vi "add datafile(SubVI).vi"(10 "字符串":string) -> (1 "ok or cancel":bool=TRUE, 2 "连接的字符串":string)   [LabVIEW 2019, in "Add Seq.lvlib"]
uses:
  Add Seq.lvlib
panel:
  in  "cancel":bool
  in  "ok":bool
  in  "operation(0:open)":T1(ring)=enum."create"
  in  "path":path
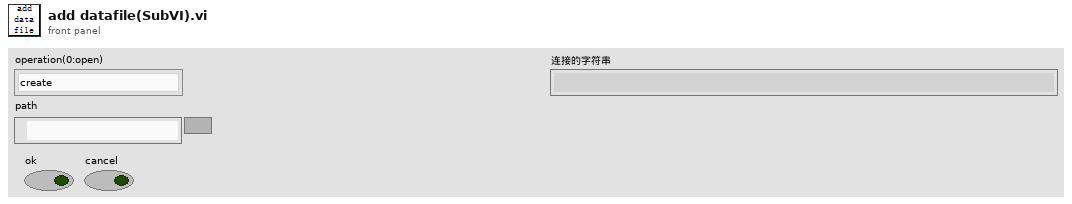
[diagram p1: front panel]
types:
  T1 = enum16{"open", "replace", "create", "open or create", "replace or create"}
  T2 = enum16{"open", "replace", "create", "open or create", "replace or create", "replace or create with confirmation"}
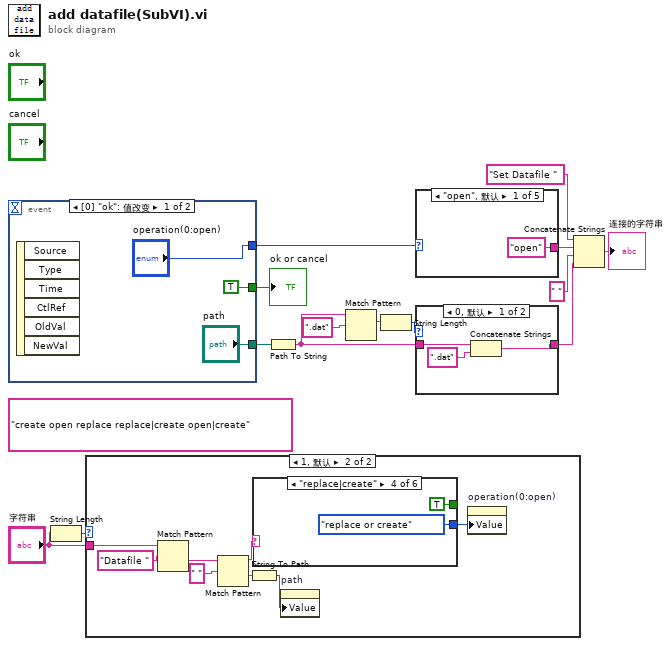
[diagram p0: block diagram]
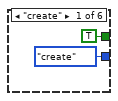
[diagram p3: hidden frame]
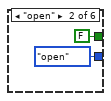
[diagram p4: hidden frame]
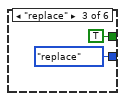
[diagram p5: hidden frame]
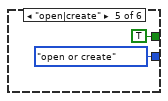
[diagram p6: hidden frame]
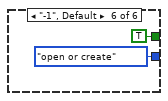
[diagram p7: hidden frame]
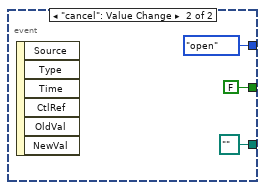
[diagram p9: hidden frame]
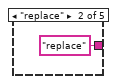
[diagram p10: hidden frame]
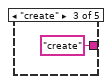
[diagram p11: hidden frame]
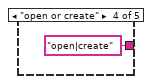
[diagram p12: hidden frame]
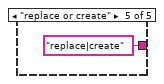
[diagram p13: hidden frame]
diagram:
  (unwired) "create open replace replace|create open|create" ("字符串")
  n1 = event shown="[0] \"ok\": 值改变" {
    selector: _ -> [_ _]
    dyn-events: _ -> [_ _]
    timeout: _ -> [_ _]
    tunnel: ["path" path "" ("path")] -> w8
    tunnel: ["operation(0:open)" T1."open" ("operation(0:open)")] -> w13
    tunnel: [TRUE FALSE] -> w9
    event "ok": Value Change {
      n2 = event-data() -> ()  [unwired: 1 in, 6 out]
    }
    event "cancel": Value Change {
      n3 = event-data() -> ()  [unwired: 1 in, 6 out]
    }
  }
  "ok or cancel" <- w9
  n4 = String Length(string="字符串") -> (length=w1:i32)
  n5 = case shown="1, 默认" w1 {
    tunnel: "字符串" -> [_ w23]
    frame 0 {
    }
    frame 1, Default {
      n6 = Match Pattern(string=w23, regular expression="Datafile " ("正则表达式")) -> (after substring=w28:string)  [unwired: 1 in, 3 out]
      n7 = Match Pattern(string=w28, regular expression=" " ("正则表达式")) -> (before substring=w22:string, after substring=w26:string)  [unwired: 1 in, 2 out]
      n8 = String To Path(string=w26) -> (path=w24:path)
      n9 = case shown="\"replace|create\"" w22 {
        tunnel: [T2."create" ("操作(0:open)") T2."open" ("操作(0:open)") T2."replace" ("操作(0:open)") T2."replace or create" ("操作(0:open)") T2."open or create" ("操作(0:open)") T2."open or create" ("操作(0:open)")] -> w25
        tunnel: [TRUE FALSE TRUE TRUE TRUE TRUE] -> _
        frame "create" {
        }
        frame "open" {
        }
        frame "replace" {
        }
        frame "replace|create" {
        }
        frame "open|create" {
        }
        frame "-1", Default {
        }
      }
      n10 = property on="path" class="Path"("Value"=w24) -> ()  [unwired: 2 in, 2 out]
      n11 = property on="operation(0:open)" class="Enum (严格)"("Value"=w25) -> ()  [unwired: 2 in, 2 out]
    }
  }
  n12 = Path To String(path=w8) -> (string=w4:string)
  n13 = Match Pattern(string=w4, regular expression=".dat" ("正则表达式")) -> (match substring=w6:string)  [unwired: 1 in, 3 out]
  n14 = String Length(string=w6) -> (length=w5:i32)
  n15 = case shown="\"open\", 默认" w13 {
    tunnel: ["open" "replace" "create" "open|create" "replace|create"] -> w12
    frame "open", Default {
    }
    frame "replace" {
    }
    frame "create" {
    }
    frame "open or create" {
    }
    frame "replace or create" {
    }
  }
  n16 = case shown="0, 默认" w5 {
    tunnel: w4 -> [w48 w49]
    tunnel: [w46 w49] -> w3
    frame 0, Default {
      n17 = Concatenate Strings(w48, ".dat" ("字符串")) -> (w46:string)
    }
    frame 4 {
    }
  }
  n18 = Concatenate Strings("Set Datafile " ("字符串"), w12, " " ("字符串"), w3) -> (→"连接的字符串":string)
